vi "Create - Enum.vi"(6 "initial timestamp":timestamp, 8 "error in (no error)":errorcluster, 9 "choices":string[](array[string]), 10 "initial index":i32) -> (0 "error out":errorcluster, 3 "NT Enum out":refnum<class "NT Enum.lvclass">)   [LabVIEW 2020, in "PV Access.lvlib" / "PV Data.lvlib" / "NT Enum.lvclass"]
uses:
  NT Enum.lvclass
  NT Enum.lvclass/NT Enum.ctl
  PV Data/PV Data.lvclass
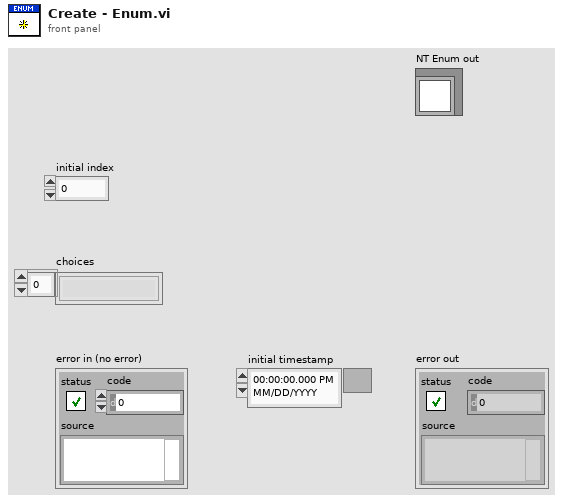
[diagram p1: front panel]
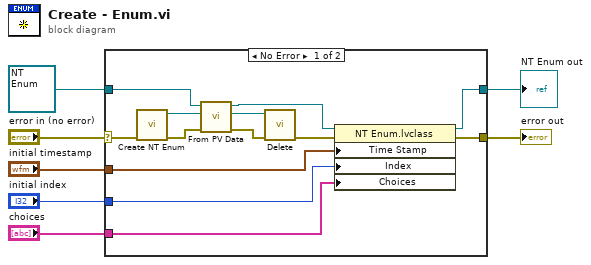
[diagram p0: block diagram]
diagram:
  n1 = case shown="No Error" "error in (no error)" {
    selector: "error in (no error)" -> [w15 w22]
    tunnel: [w19 w22] -> w6
    tunnel: [w20 w21] -> w4
    tunnel: refnum<class "NT Enum.lvclass"> refnum ("NT Enum in") -> [w12 w21]
    tunnel: "initial index" -> [w17 _]
    tunnel: "choices" -> [w16 _]
    tunnel: "initial timestamp" -> [w18 _]
    frame No Error {
      n2 = call "Create NT Enum.vi"("error in"=w15) -> ("error out"=w13:errorcluster, "PV Data out"=w14:refnum<class "PV Data.lvclass">)  [unwired: 9 in]
      n3 = call-dynamic "From PV Data.vi"("error in"=w13, "PV data in"=w14, "Base Interface in"=w12) -> ("error out"=w11:errorcluster, "PV data out"=w10:refnum<class "PV Data.lvclass">, "Base Interface out"=w9:refnum<class "NT Enum.lvclass">)  [unwired: 6 in]
      n4 = call "Delete.vi"("error in (no error)"=w11, "PV Data in"=w10) -> ("error out"=w8:errorcluster)  [unwired: 9 in]
      n5 = property class="NT Enum.lvclass"(reference=w9, error in=w8, "Time Stamp"=w18, "Index"=w17, "Choices"=w16) -> (reference out=w20:refnum<class "NT Enum.lvclass">, error out=w19:errorcluster)
    }
    frame Error {
    }
  }
  "error out" <- w6
  "NT Enum out" <- w4
